vi "Test Time UI.vi"() -> ()   [LabVIEW 2013]
panel:
  in  "Boolean":bool
  in  "Time Stamp":timestamp
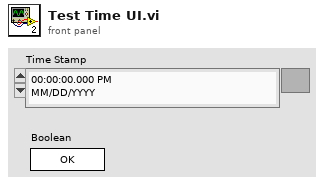
[diagram p1: front panel]
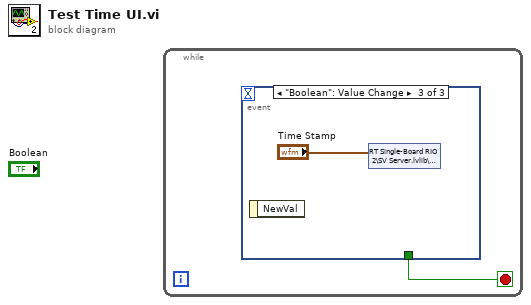
[diagram p0: block diagram]
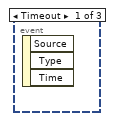
[diagram p2: hidden frame]
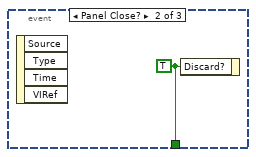
[diagram p3: hidden frame]
diagram:
  n1 = while {
    stop <- w1 stop-if-true
    n2 = event shown="[2] \"Boolean\": Value Change" {
      selector: _ -> [_ _ _]
      dyn-events: _ -> [_ _ _]
      timeout: _ -> [_ _ _]
      tunnel: [_ w2 _] -> w1
      event Timeout {
        n3 = event-data() -> ()  [unwired: 1 in, 3 out]
      }
      event Panel Close? {
        w2 = TRUE ("Discard?")
        n4 = event-data() -> ()  [unwired: 1 in, 4 out]
        n5 = event-data("Discard?"=w2) -> ()  [unwired: 1 in, 1 out]
      }
      event "Boolean": Value Change {
        n6 = event-data() -> ()  [unwired: 1 in, 1 out]
        n7 = shared-variable "RT Single-Board RIO 2\\SV Server.lvlib\\Time"("Time Stamp") -> ()  [unwired: 1 in, 1 out]
      }
    }
  }
